vi "PH_OceanOpticsSpectrometer.evt call Set Display.vi"(0 "i ref in":refnum<vi>, 2 "Instance":string="N/A", 3 "Integration Time [ms]":dbl=50.0, 4 "Center":dbl=1054.0, 5 "error in (no error)":errorcluster) -> (14 "i ref out":refnum<vi>, 19 "error out":errorcluster)   [LabVIEW 2014, in "PH_OceanOpticsSpectrometer.lvlib"]
doc: "This VI sends a comand by a simple call."
uses:
  PH_OceanOpticsSpectrometer.lvlib
  CS_Core/CSSystem/CoreLib/CoreLib.double 2 byte array.vi
  CS_Core/CSSystem/CoreLib/CoreLib.lvlib
  CS_Core/BaseProcess/BaseProcess.lvlib
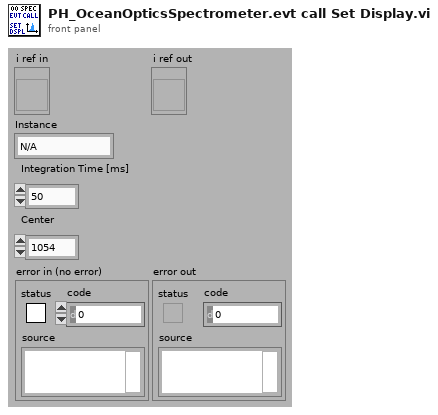
[diagram p1: front panel]
types:
  T1 = typedef "CoreDefs.rawDataType.ctl" = i8[]
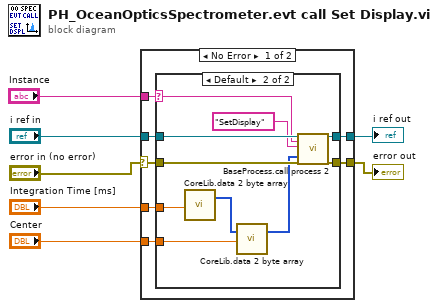
[diagram p0: block diagram]
diagram:
  n1 = case shown="No Error" "error in (no error)" {
    selector: "error in (no error)" -> [w10 w27]
    tunnel: [w14 w28] -> w3
    tunnel: [w13 w27] -> w4
    tunnel: "i ref in" -> [w12 w28]
    tunnel: "Instance" -> [w11 _]
    tunnel: "Integration Time [ms]" -> [w9 _]
    tunnel: "Center" -> [w8 _]
    frame No Error {
      n2 = case shown="Default" w11 {
        selector: w11 -> [_ w21]
        tunnel: [w16 w26] -> w14
        tunnel: [w15 w25] -> w13
        tunnel: w12 -> [w16 w24]
        tunnel: w10 -> [w15 w23]
        tunnel: w9 -> [_ w20]
        tunnel: w8 -> [_ w19]
        frame "N/A" {
        }
        frame Default {
          n3 = call-poly "CoreLib.data 2 byte array.vi"("f64"=w20) -> ("byteArray out"=w18:T1)  [unwired: 18 in]
          n4 = call-poly "CoreLib.data 2 byte array.vi"("byteArray"=w18, "f64"=w19) -> ("byteArray out"=w17:T1)  [unwired: 17 in]
          n5 = call "BaseProcess.call process 2.vi"("i ref in"=w24, "Object"=w21, "Selector"="SetDisplay", "Data"=w17, "error in (no error)"=w23) -> ("i ref out"=w26:refnum<vi>, "error out"=w25:errorcluster)  [unwired: 13 in]
        }
      }
    }
    frame Error {
    }
  }
  "error out" <- w4
  "i ref out" <- w3
